vi "Kelvin Functions ke.vi"(2 "n":i32, 3 "x":dbl format="%.2f") -> (1 "ker(x) + kei(x)i":cdb format="%.2f")   [LabVIEW 2017, in "NI_Gmath.lvlib"]
doc: "Computes the complex Kelvin function of the second kind."
uses:
  <vilib>/gmath/NI_Gmath.lvlib
  <resource>/lvanlys.dll
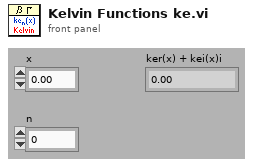
[diagram p1: front panel]
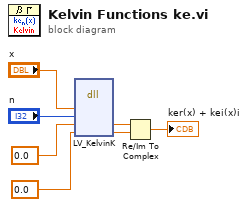
[diagram p0: block diagram]
diagram:
  n1 = dll-call lib="e:/builds/penguin/labview/branches/2017/dev/dist/resource/lvanlys.*" fn="LV_KelvinK"("x"="x", "n"="n", "ker"=0.0 ("ber"), "kei"=0.0 ("bei")) -> ("ker"=w3:dbl, "kei"=w2:dbl)  [unwired: 6 in, 2 out]
  n2 = Re/Im To Complex(1:w2, 2:w3) -> (0:→"ker(x) + kei(x)i":cdb)
